vi "RecordPlayersMoves.vi"(8 "error in (no error)":errorcluster, 9 "Player2Move":T1, 10 "Player1Move":T1, 11 "GameRecorder in":refnum<class "GameRecorder.lvclass">) -> (0 "error out":errorcluster, 3 "GameRecorder out":refnum<class "GameRecorder.lvclass">)   [LabVIEW 2015, in "TronviewGame.lvlib" / "GameRecorder.lvclass"]
uses:
  GameRecorder.lvclass
  TronVIEWBotAPI/MovementDirection.ctl
  GameRecorder.lvclass/GameRecorder.ctl
  TronVIEWBotAPI/TronVIEWBotAPI.lvlib
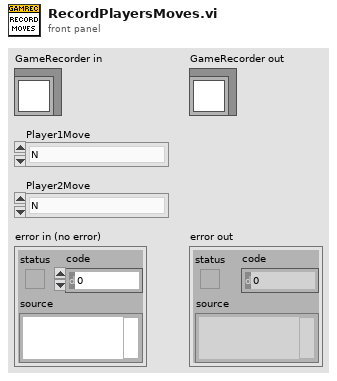
[diagram p1: front panel]
types:
  T1 = typedef "TronVIEWBotAPI.lvlib/MovementDirection.ctl" = enum16{"N", "S", "W", "E"}
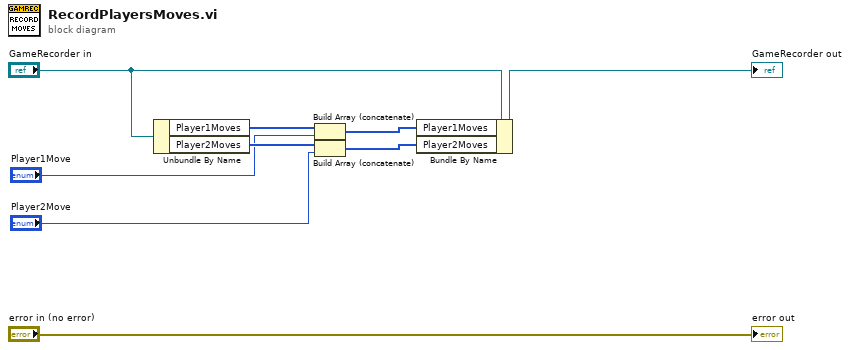
[diagram p0: block diagram]
diagram:
  n1 = Unbundle By Name("GameRecorder in") -> ("Player1Moves"=w6:T1[], "Player2Moves"=w5:T1[])
  n2 = Build Array (concatenate)(w6, "Player1Move") -> (w4:T1[])
  n3 = Build Array (concatenate)(w5, "Player2Move") -> (w3:T1[])
  n4 = Bundle By Name(cluster="GameRecorder in", "Player1Moves"=w4, "Player2Moves"=w3) -> (→"GameRecorder out":refnum<class "GameRecorder.lvclass">)
  "error out" <- "error in (no error)"
